vi "ExPluginRunVi.vi"(0 "VI Refnum":refnum<vi>, 1 "Controls Name":string[](array[string]), 2 "Values":variant[](array[variant]), 5 "error in":errorcluster, 6 "Front Panel Behavior":T1(ring)=enum."Floating", 7 "Wait Until Done":bool, 8 "ShowFP":bool=TRUE, 9 "LoadVariableIf RUN":bool, 11 "DoNotCentered If RUN":bool, 13 "Front Panel Window:Is Frontmost":bool) -> (19 "error out":errorcluster)   [LabVIEW 2018]
panel:
  # "Открывает VI по ссылке. Если уже открыта, то выносит на передний край.\nПередает ссылку на базу данных, так же возможно передать в VI массив контролов \nи их значения"
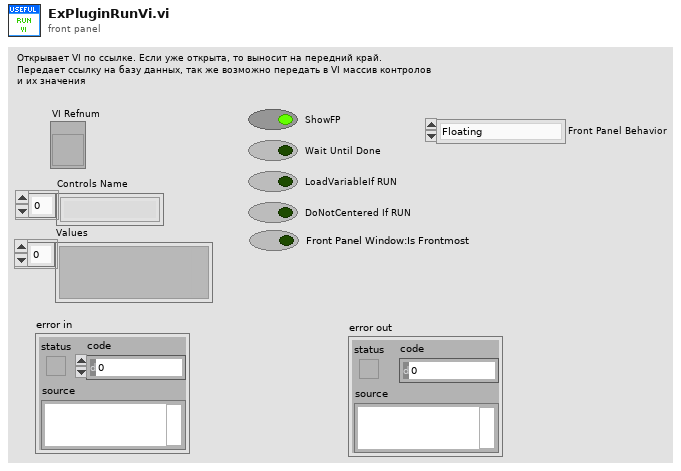
[diagram p1: front panel]
types:
  T1 = enum32{"Invalid", "Default", "Floating", "Floating/Auto-Hide", "Modal"}
  T2 = enum32{"Bad", "Idle", "Run top level", "Running"}
  T3 = enum32{"Invalid", "Standard", "Closed", "Hidden", "Minimized", "Maximized"}
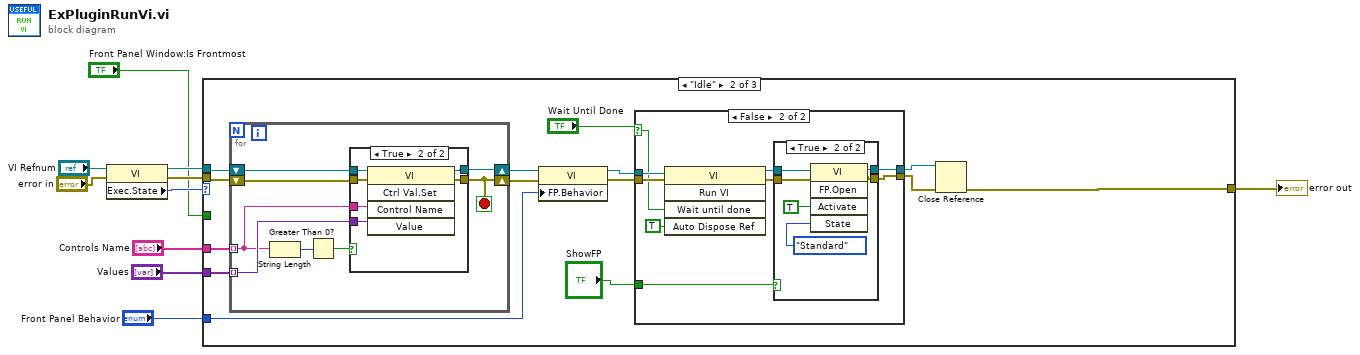
[diagram p0: block diagram]
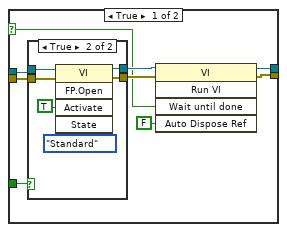
[diagram p3: hidden frame]
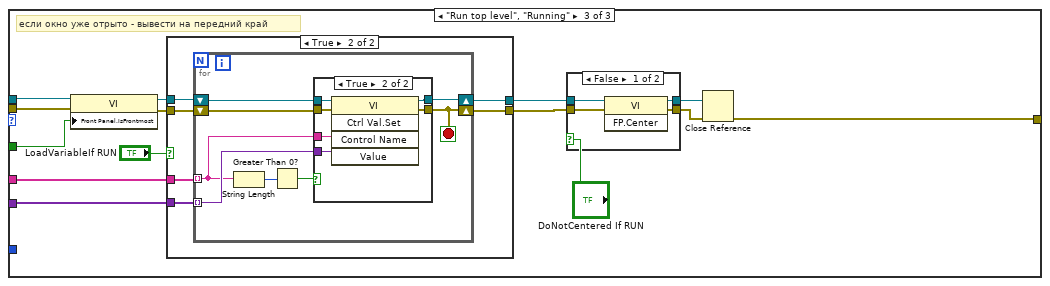
[diagram p7: hidden frame]
diagram:
  n1 = property class="VI"(reference="VI Refnum", error in="error in") -> (reference out=w8:refnum<vi>, error out=w7:errorcluster, "Exec.State"=w9:T2)
  n2 = case shown="\"Idle\"" w9 {
    tunnel: w8 -> [_ w20 w89]
    tunnel: w7 -> [w11 w19 w88]
    tunnel: "Controls Name" -> [_ w25 w86]
    tunnel: "Values" -> [_ w24 w85]
    tunnel: [w11 w21 w87] -> w3
    tunnel: "Front Panel Behavior" -> [_ w14 _]
    tunnel: "Front Panel Window:Is Frontmost" -> [_ _ w76]
    frame "Bad", Default {
    }
    frame "Idle" {
      n3 = for {
        shift-right: [w66] -> w22
        shift-left: w19 -> [w67]
        tunnel: w25 -> [w64] mode=indexing
        tunnel: w24 -> [w65] mode=indexing
        shift-right: [w60] -> w23
        shift-left: w20 -> [w61]
        stop <- w66 stop-if-true
        n4 = String Length(string=w64) -> (length=w63:i32)
        n5 = Greater Than 0?(x=w63) -> (x > 0?=w62:bool)
        n6 = case shown="True" w62 {
          tunnel: w61 -> [w68 w75]
          tunnel: w67 -> [w69 w74]
          tunnel: [w69 w73] -> w66
          tunnel: w64 -> [_ w72]
          tunnel: w65 -> [_ w71]
          tunnel: [w68 w70] -> w60
          frame False {
          }
          frame True {
            n7 = invoke class="VI" method="Ctrl Val.Set"(reference=w75, error in=w74, "Control Name"=w72, "Value"=w71) -> (reference out=w70:refnum<vi>, error out=w73:errorcluster)  [unwired: 1 in, 3 out]
          }
        }
      }
      n8 = property class="VI"(reference=w23, error in=w22, "FP.Behavior"=w14) -> (reference out=w18:refnum<vi>, error out=w17:errorcluster)
      n9 = case shown="False" "Wait Until Done" {
        selector: "Wait Until Done" -> [w26 w43]
        tunnel: w18 -> [w33 w50]
        tunnel: w17 -> [w32 w49]
        tunnel: [w29 w46] -> w12
        tunnel: [w28 w45] -> w13
        tunnel: "ShowFP" -> [w34 w44]
        frame True {
          n10 = case shown="True" w34 {
            tunnel: [w36 w42] -> w31
            tunnel: [w35 w41] -> w30
            tunnel: w32 -> [w35 w37]
            tunnel: w33 -> [w36 w38]
            frame False {
            }
            frame True {
              n11 = invoke class="VI" method="FP.Open"(reference=w38, error in=w37, "Activate"=TRUE ("Activate?"), "State"=T3."Standard") -> (reference out=w42:refnum<vi>, error out=w41:errorcluster)  [unwired: 1 in, 3 out]
            }
          }
          n12 = invoke class="VI" method="Run VI"(reference=w31, error in=w30, "Wait until done"=w26, "Auto Dispose Ref"=FALSE ("Auto Dispose Reference")) -> (reference out=w28:refnum<vi>, error out=w29:errorcluster)  [unwired: 1 in, 3 out]
        }
        frame False {
          n13 = invoke class="VI" method="Run VI"(reference=w50, error in=w49, "Wait until done"=w43, "Auto Dispose Ref"=TRUE ("Auto Dispose Reference")) -> (reference out=w48:refnum<vi>, error out=w47:errorcluster)  [unwired: 1 in, 3 out]
          n14 = case shown="True" w44 {
            tunnel: [w53 w59] -> w45
            tunnel: [w52 w58] -> w46
            tunnel: w47 -> [w52 w54]
            tunnel: w48 -> [w53 w55]
            frame False {
            }
            frame True {
              n15 = invoke class="VI" method="FP.Open"(reference=w55, error in=w54, "Activate"=TRUE ("Activate?"), "State"=T3."Standard") -> (reference out=w59:refnum<vi>, error out=w58:errorcluster)  [unwired: 1 in, 3 out]
            }
          }
        }
      }
      n16 = Close Reference(reference=w13, error in (no error)=w12) -> (error out=w21:errorcluster)
    }
    frame "Run top level", "Running" {
      # "если окно уже отрыто - вывести на передний край"
      n17 = property class="VI"(reference=w89, error in=w88, "Front Panel.IsFrontmost"=w76) -> (reference out=w83:refnum<vi>, error out=w82:errorcluster)
      n18 = case shown="True" "LoadVariableIf RUN" {
        tunnel: w83 -> [w97 w103]
        tunnel: w82 -> [w96 w102]
        tunnel: [w97 w101] -> w79
        tunnel: [w96 w100] -> w78
        tunnel: w86 -> [_ w99]
        tunnel: w85 -> [_ w98]
        frame False {
        }
        frame True {
          n19 = for {
            shift-right: [w110] -> w100
            shift-left: w102 -> [w111]
            tunnel: w99 -> [w108] mode=indexing
            tunnel: w98 -> [w109] mode=indexing
            shift-right: [w104] -> w101
            shift-left: w103 -> [w105]
            stop <- w110 stop-if-true
            n20 = String Length(string=w108) -> (length=w107:i32)
            n21 = Greater Than 0?(x=w107) -> (x > 0?=w106:bool)
            n22 = case shown="True" w106 {
              tunnel: w105 -> [w112 w119]
              tunnel: w111 -> [w113 w118]
              tunnel: [w113 w117] -> w110
              tunnel: w108 -> [_ w116]
              tunnel: w109 -> [_ w115]
              tunnel: [w112 w114] -> w104
              frame False {
              }
              frame True {
                n23 = invoke class="VI" method="Ctrl Val.Set"(reference=w119, error in=w118, "Control Name"=w116, "Value"=w115) -> (reference out=w114:refnum<vi>, error out=w117:errorcluster)  [unwired: 1 in, 3 out]
              }
            }
          }
        }
      }
      n24 = case shown="False" "DoNotCentered If RUN" {
        tunnel: [w93 w95] -> w81
        tunnel: [w92 w94] -> w80
        tunnel: w79 -> [w91 w95]
        tunnel: w78 -> [w90 w94]
        frame False {
          n25 = invoke class="VI" method="FP.Center"(reference=w91, error in=w90) -> (reference out=w93:refnum<vi>, error out=w92:errorcluster)  [unwired: 1 in, 1 out]
        }
        frame True {
        }
      }
      n26 = Close Reference(reference=w81, error in (no error)=w80) -> (error out=w87:errorcluster)
    }
  }
  "error out" <- w3
